vi "Prepare RProp.vi"(11 "Neural Network In":refnum<class "Neural Network.lvclass">) -> (2 "Teach Coef Buffer":T1[](array[typedef]), 3 "Gradient Buffer":T1[](array[typedef]))   [LabVIEW 2015, in "Neural Network.lvclass"]
uses:
  Neural Network.lvclass
  Types/2D Array.ctl
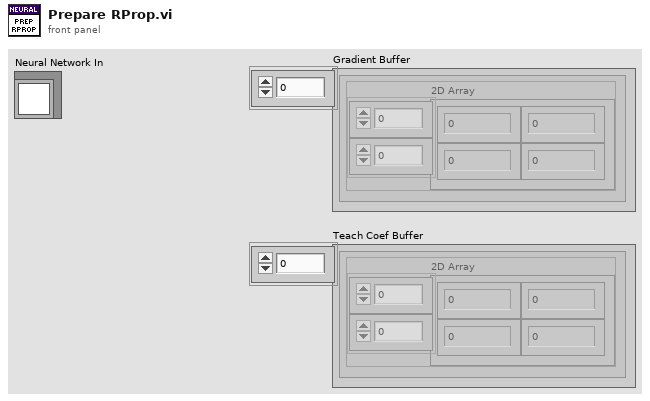
[diagram p1: front panel]
types:
  T1 = typedef "Neural Network.lvclass/2D Array.ctl" = cluster{"2D Array":sgl[][]}
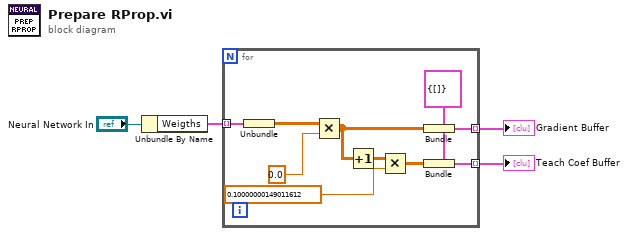
[diagram p0: block diagram]
diagram:
  n1 = Unbundle By Name("Neural Network In") -> ("Weigths"=w1:T1[])
  n2 = for {
    tunnel: w1 -> [w14] mode=indexing
    tunnel: [w11] -> w3 mode=indexing
    tunnel: [w5] -> w4 mode=indexing
    w10 = T1 {"2D Array"=[]}
    n3 = Unbundle(w14) -> ("2D Array"=w12:sgl[][])
    n4 = Multiply(x=w12, y=sgl 0.0) -> (x*y=w8:sgl[][])
    n5 = Increment(x=w8) -> (x+1=w9:sgl[][])
    n6 = Multiply(x=w9, y=sgl 0.1) -> (x*y=w6:sgl[][])
    n7 = Bundle(cluster=w10, "2D Array"=w8) -> (w11:T1)
    n8 = Bundle(cluster=w10, "2D Array"=w6) -> (w5:T1)
  }
  "Teach Coef Buffer" <- w4
  "Gradient Buffer" <- w3
